vi "PicoScope5000aIsReady.vi"(8 "error in (no error)":errorcluster, 11 "handle in":i16) -> (0 "error out":errorcluster, 3 "handle out":i16, 6 "ready":i16=1)   [LabVIEW 2020]
doc: "Calls ps5000aIsReady"
uses:
  ps5000a.dll
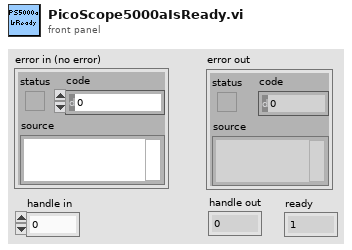
[diagram p1: front panel]
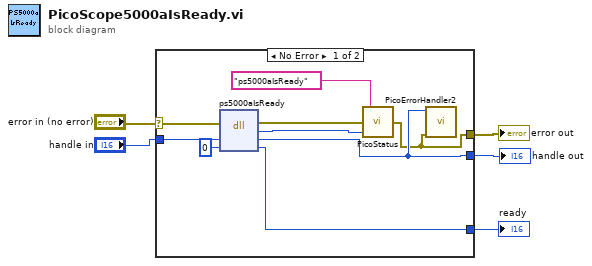
[diagram p0: block diagram]
diagram:
  n1 = case shown="No Error" "error in (no error)" {
    selector: "error in (no error)" -> [w13 w15]
    tunnel: "handle in" -> [w14 w16]
    tunnel: [w10 w16] -> w5
    tunnel: [w7 w15] -> w4
    tunnel: [w6 _] -> w3
    frame No Error {
      n2 = dll-call lib="ps5000a.dll" fn="ps5000aIsReady" ("ps3000.dll:_ps3000_open_unit@0")(error in=w13, "handle"=w14, "ready"=i16 0) -> (error out=w12:errorcluster, "PICO_STATUS"=w8:u32, "handle"=w10:i16, "ready"=w6:i16)  [unwired: 2 in, 1 out]
      n3 = call "PicoStatus.vi"("PICO STATUS"=w8, "error in"=w12, "source"="ps5000aIsReady") -> ("error out"=w7:errorcluster)
      n4 = call "PicoErrorHandler2.vi"("error in (no error)"=w7, "handle In"=w10) -> ()  [unwired: 9 in, 1 out]
    }
    frame Error {
    }
  }
  "error out" <- w4
  "handle out" <- w5
  "ready" <- w3
